vi "IntensityProfileAlongCoord.vi"(8 "error in (no error)":errorcluster, 9 "Coord":cluster{"X Centroid":sgl, "Y Centroid":sgl}={"X Centroid"=366.21008, "Y Centroid"=248.15193} {"Y Centroid" format="%.2f"; "X Centroid" format="%.2f"}, 11 "Image Src":T1) -> (0 "error out":errorcluster, 1 "Y Intensity (U8)":u8[](array[numeric]), 2 "X Intensity (U8)":u8[](array[numeric]))   [LabVIEW 2013]
uses:
  <vilib>/vision/Image Controls.llb/IMAQ Image.ctl
  <vilib>/vision/NI_Vision_Development_Module.lvlib
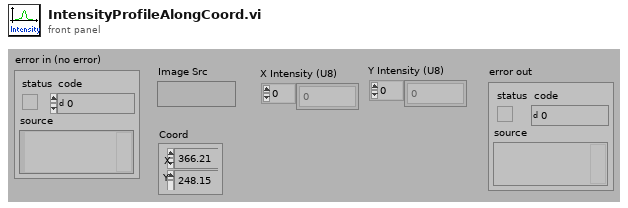
[diagram p1: front panel]
types:
  T1 = typedef "IMAQ Image.ctl" = refnum<image>
  T2 = typedef "Image Type" = u32
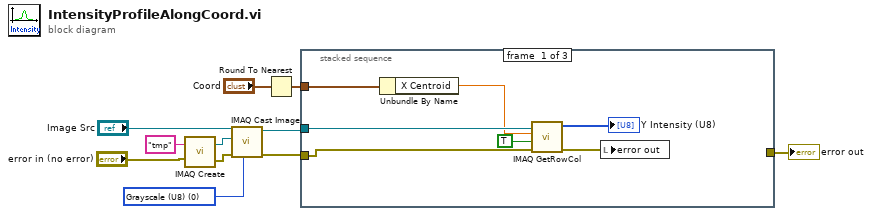
[diagram p0: block diagram]
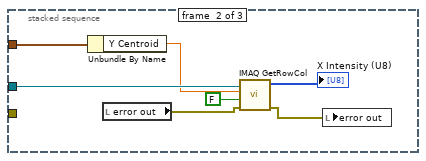
[diagram p2: hidden frame]
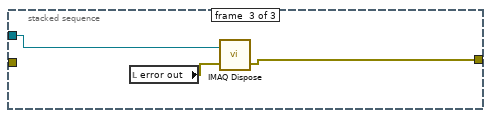
[diagram p3: hidden frame]
diagram:
  w11 = T2 0 items=["Grayscale (U8)", "Grayscale (I16)", "Grayscale (SGL)", "Complex (CSG)", "RGB (U32)", "HSL (U32)", "RGB (U64)", "Grayscale (U16)"] ("Image Type")
  n1 = call "IMAQ Create"("Image Name"="tmp", "error in (no error)"="error in (no error)") -> ("New Image"=w4:T1, "error out"=w3:errorcluster)  [unwired: 2 in, 1 out]
  n2 = call "IMAQ Cast Image"("Image Type"=w11, "error in (no error)"=w3, "Image Dst"=w4, "Image Src"="Image Src") -> ("error out"=w9:errorcluster, "Image Dst Out"=w10:T1)  [unwired: 2 in, 4 out]
  n3 = Round To Nearest(number="Coord") -> (nearest integer value=w7:cluster{"X Centroid":sgl, "Y Centroid":sgl})
  n4 = stacked-sequence {
    tunnel: w10 -> [w18 w25 w28]
    tunnel: w9 -> [w13 _ _]
    tunnel: w7 -> [w15 w23 _]
    tunnel: [_ _ w27] -> w5
    frame #0 {
      n5 = Unbundle By Name(w15) -> ("X Centroid"=w14:sgl)
      n6 = call "IMAQ GetRowCol"("Image"=w18, "Number"=w14, "Row / Column (Row)"=TRUE, "error in (no error)"=w13) -> ("Pixels (U8)"=→"Y Intensity (U8)":u8[], "error out"=w17:errorcluster)  [unwired: 5 out]
      n7 = local write "error out"(w17) -> ()
    }
    frame #1 {
      n8 = Unbundle By Name(w23) -> ("Y Centroid"=w22:sgl)
      n9 = local read "error out"() -> (w24:errorcluster)
      n10 = call "IMAQ GetRowCol"("Image"=w25, "Number"=w22, "Row / Column (Row)"=FALSE, "error in (no error)"=w24) -> ("Pixels (U8)"=→"X Intensity (U8)":u8[], "error out"=w19:errorcluster)  [unwired: 5 out]
      n11 = local write "error out"(w19) -> ()
    }
    frame #2 {
      n12 = local read "error out"() -> (w26:errorcluster)
      n13 = call "IMAQ Dispose"("Image"=w28, "error in (no error)"=w26) -> ("error out"=w27:errorcluster)  [unwired: 1 in, 3 out]
    }
  }
  "error out" <- w5
